vi "Generate Error.vi"(7 "Mode":T1(ring), 8 "error in (no error)":errorcluster, 11 "Method Result In":refnum<class "Method Result.lvclass">) -> (0 "error out":errorcluster, 3 "Method Result Out":refnum<class "Method Result.lvclass">)   [LabVIEW 2020, in "Method Result.lvclass"]
uses:
  Method Result.lvclass
  Assertion Result/Public/TypeDefs/Status.ctl
  Method Result.lvclass/Method Result.ctl
  Assertion Result/Assertion Result.lvclass
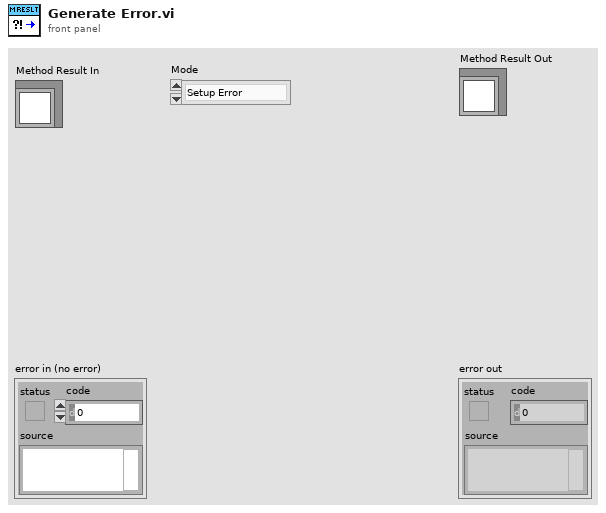
[diagram p1: front panel]
types:
  T1 = enum16{"Setup Error", "Teardown Error", "Broken", "Test Method Error"}
  T2 = typedef "Assertion Result.lvclass/Status.ctl" = enum16{"Pass", "Fail", "Error", "Skipped", "Setup Error", "Broken", "Teardown Error"}
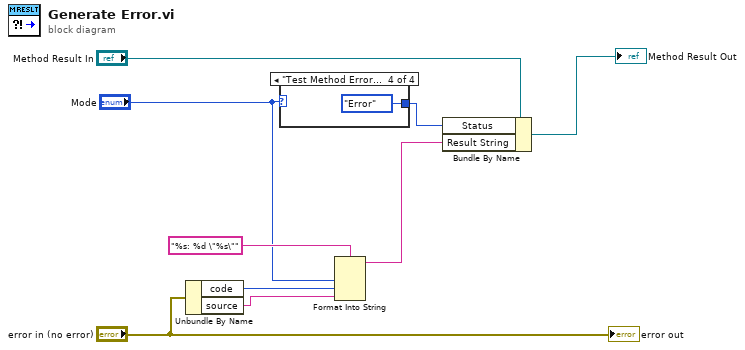
[diagram p0: block diagram]
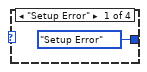
[diagram p2: hidden frame]
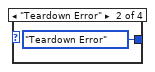
[diagram p3: hidden frame]
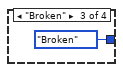
[diagram p4: hidden frame]
diagram:
  n1 = Unbundle By Name("error in (no error)") -> ("code"=w5:i32, "source"=w4:string)
  n2 = case shown="\"Test Method Error\"" "Mode" {
    tunnel: [Status."Setup Error" ("Status") Status."Teardown Error" ("Status") Status."Broken" ("Status") Status."Error" ("Status")] -> w8
    frame "Setup Error" {
    }
    frame "Teardown Error" {
    }
    frame "Broken" {
    }
    frame "Test Method Error" {
    }
  }
  n3 = Format Into String(format string="%s: %d \"%s\"", "Mode", w5, w4) -> (resulting string=w1:string)  [unwired: 2 in, 1 out]
  n4 = Bundle By Name(cluster="Method Result In", "Status"=w8, "Result String"=w1) -> (→"Method Result Out":refnum<class "Method Result.lvclass">)
  "error out" <- "error in (no error)"
